vi "Read configuration.vi"(8 "error in":errorcluster, 11 "Custom Controller Module editor node in":refnum<class "Custom Controller Module editor node.lvclass">) -> (0 "error out":errorcluster, 2 "configuration":refnum<class "NISE_CEF_serializable configuration.lvclass">, 3 "Custom Controller Module editor node out":refnum<class "Custom Controller Module editor node.lvclass">)   [LabVIEW 2013, in "Custom Controller Module editor node.lvclass"]
uses:
  Custom Controller Module editor node.lvclass
  <vilib>/NI/Configuration Framework/serializable configuration/NISE_CEF_serializable configuration.lvclass
  Custom Controller Module editor node.lvclass/Custom Controller Module editor node.ctl
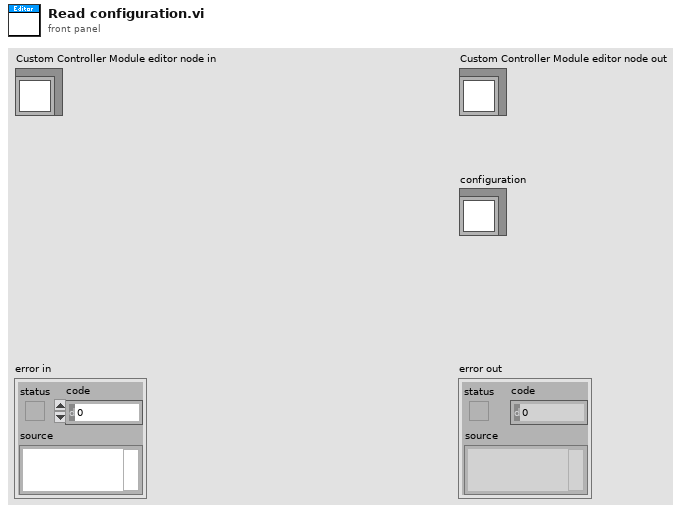
[diagram p1: front panel]
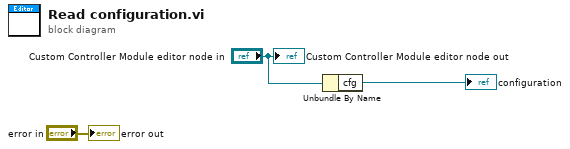
[diagram p0: block diagram]
diagram:
  n1 = Unbundle By Name("Custom Controller Module editor node in") -> ("cfg"=→"configuration":refnum<class "Custom Controller Module configuration.lvclass">)
  "error out" <- "error in"
  "Custom Controller Module editor node out" <- "Custom Controller Module editor node in"
